vi "MyRIO Lidar Class Data.vi"() -> ()   [LabVIEW 2016]
panel:
  out "MyRio Lidar class data":T1
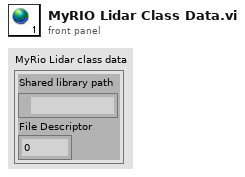
[diagram p1: front panel]
types:
  T1 = cluster{"Shared library path":path, "File Descriptor":i32}
diagram:
